vi "FindUSBDevice.vi"(11 "DevSNin":string) -> (0 "DevSN":string, 1 "BOARD_INFO":T1, 2 "DevNum":i32=-1, 3 "Total":u32, 5 "SNs":string[](array[string]))   [LabVIEW 2011]
uses:
  data/ControlCAN.dll
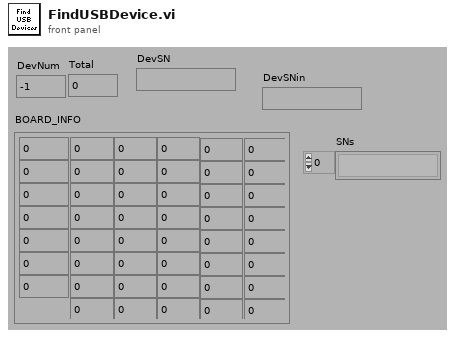
[diagram p1: front panel]
types:
  T1 = cluster{"hw_Version":u16, "fw_Version":u16, "dr_Version":u16, "in_Version":u16, "irq_Num":u16, "can_Num":u8, "reserved":u8, "sSN0":u8, "sSN1":u8, "sSN2":u8, "sSN3":u8, "sSN4":u8, "sSN5":u8, "sSN6":u8, "sSN7":u8, "shwT0":u8, "shwT1":u8, "shwT2":u8, "shwT3":u8, "shwT4":u8, "shwT5":u8, "shwT6":u8, "shwT7":u8, "shwT8":u8, "shwT9":u8, "shwT10":u8, "shwT11":u8, "shwT12":u8, "shwT13":u8, "shwT14":u8, "shwT15":u8, "sUSN0":u8, "sUSN1":u8, "sUSN2":u8, "sUSN3":u8, "sUSN4":u8, "sUSN5":u8, "sUSN6":u8, "sUSN7":u8, "sUSN8":u8, "sUSN9":u8, "sUSN10":u8, "sUSN11":u8, "sUSN12":u8, "sUSN13":u8, "sUSN14":u8, "sUSN15":u8}
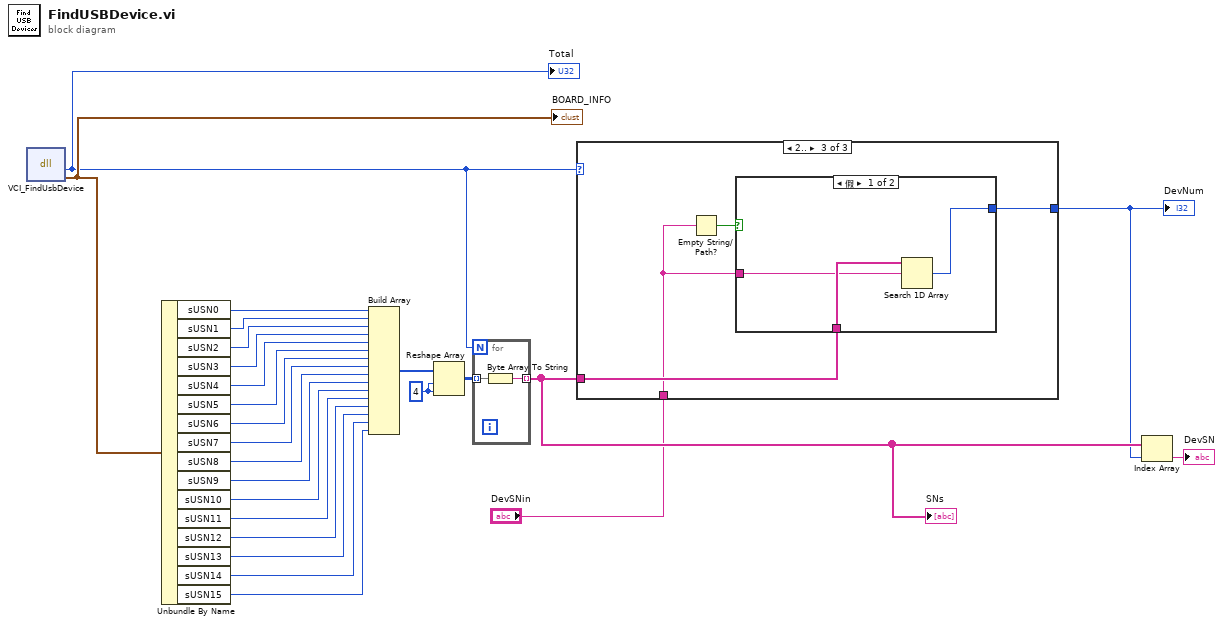
[diagram p0: block diagram]
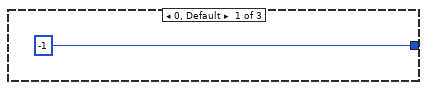
[diagram p2: hidden frame]
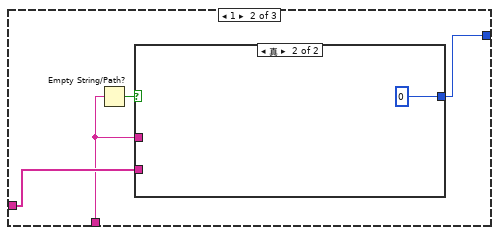
[diagram p3: hidden frame]
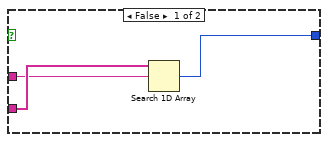
[diagram p4: hidden frame]
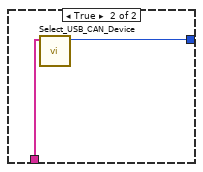
[diagram p5: hidden frame]
diagram:
  w24 = 4 ("维数大小")
  n1 = dll-call lib="PTH1Yabs D\t董海成\t上位机2.进行中USB-CAN Tool\t兼容ZLGdataControlCAN.dll" fn="VCI_FindUsbDevice"() -> ("返回类型"=w5:u32, "BOARD_INFO"=w6:T1)  [unwired: 4 in, 2 out]
  "Total" <- w5
  "BOARD_INFO" <- w6
  n2 = Unbundle By Name(w6) -> ("sUSN0"=w7:u8, "sUSN1"=w8:u8, "sUSN2"=w9:u8, "sUSN3"=w10:u8, "sUSN4"=w11:u8, "sUSN5"=w12:u8, "sUSN6"=w13:u8, "sUSN7"=w14:u8, "sUSN8"=w15:u8, "sUSN9"=w16:u8, "sUSN10"=w17:u8, "sUSN11"=w18:u8, "sUSN12"=w19:u8, "sUSN13"=w20:u8, "sUSN14"=w21:u8, "sUSN15"=w22:u8)
  n3 = Build Array(w7, w8, w9, w10, w11, w12, w13, w14, w15, w16, w17, w18, w19, w20, w21, w22) -> (w23:u8[])
  n4 = Reshape Array(w23, w24, w24) -> (w25:u8[][])
  n5 = for {
    N: w5 -> [_]
    tunnel: w25 -> [w27] mode=indexing
    tunnel: [w26] -> w4 mode=indexing
    n6 = Byte Array To String(unsigned byte array=w27) -> (string=w26:string)
  }
  "SNs" <- w4
  n7 = case shown="2.." w5 {
    tunnel: [-1 ("DevNum") w31 w40] -> w3
    tunnel: w4 -> [_ w30 w39]
    tunnel: "DevSNin" -> [_ w29 w37]
    frame 0, Default {
    }
    frame 1 {
      n8 = Empty String/Path?(string/path=w29) -> (empty?=w32:bool)
      n9 = case shown="真" w32 {
        tunnel: [w33 0 ("DevNum")] -> w31
        tunnel: w30 -> [w35 _]
        tunnel: w29 -> [w34 _]
        frame False {
          n10 = Search 1D Array(1D array=w35, element=w34) -> (index of element=w33:i32)  [unwired: 1 in]
        }
        frame True {
        }
      }
    }
    frame 2.. {
      n11 = Empty String/Path?(string/path=w37) -> (empty?=w38:bool)
      n12 = case shown="假" w38 {
        tunnel: [w41 w45] -> w40
        tunnel: w39 -> [w43 w44]
        tunnel: w37 -> [w42 _]
        frame False {
          n13 = Search 1D Array(1D array=w43, element=w42) -> (index of element=w41:i32)  [unwired: 1 in]
        }
        frame True {
          n14 = call "Select_USB_CAN_Device.vi"("DevNames"=w44) -> ("DevNum"=w45:i32)  [unwired: 10 in]
        }
      }
    }
  }
  "DevNum" <- w3
  n15 = Index Array(array=w4, index=w3) -> (element=→"DevSN":string)
